vi "Path_Function_Deviation.vi"(10 "Function In":string, 11 "Path Points In":T1(array[cluster])) -> (3 "Path Points Out":T1(array[cluster]))   [LabVIEW 2019]
uses:
  <vilib>/gmath/NI_Gmath.lvlib
panel:
  out "X":dbl[][](graph)
  out "Y":dbl[][](graph)
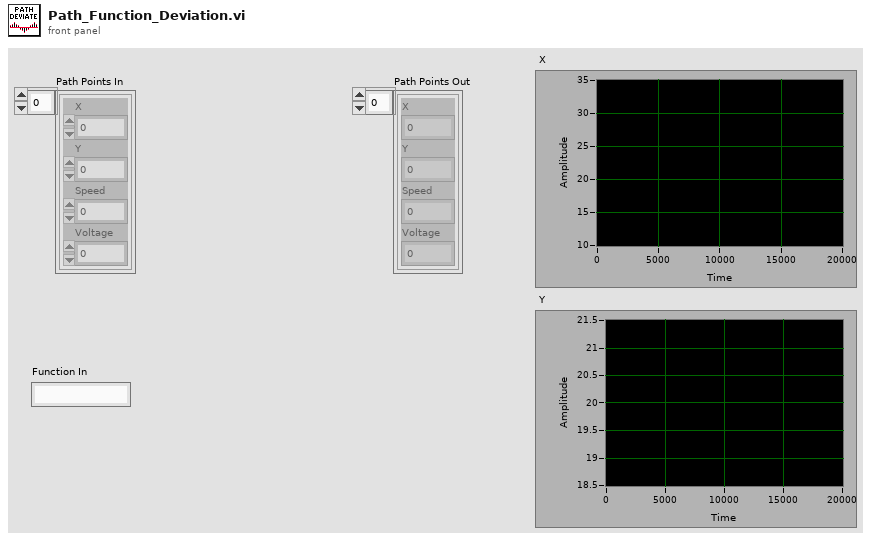
[diagram p1: front panel]
types:
  T1 = cluster{"X":dbl, "Y":dbl, "Speed":dbl, "Voltage":dbl}[]
  T2 = cluster{"X":dbl, "Y":dbl, "Speed":dbl, "Voltage":dbl}
  T3 = cluster{"X":bool, "Y":bool, "Speed":bool, "Voltage":bool}
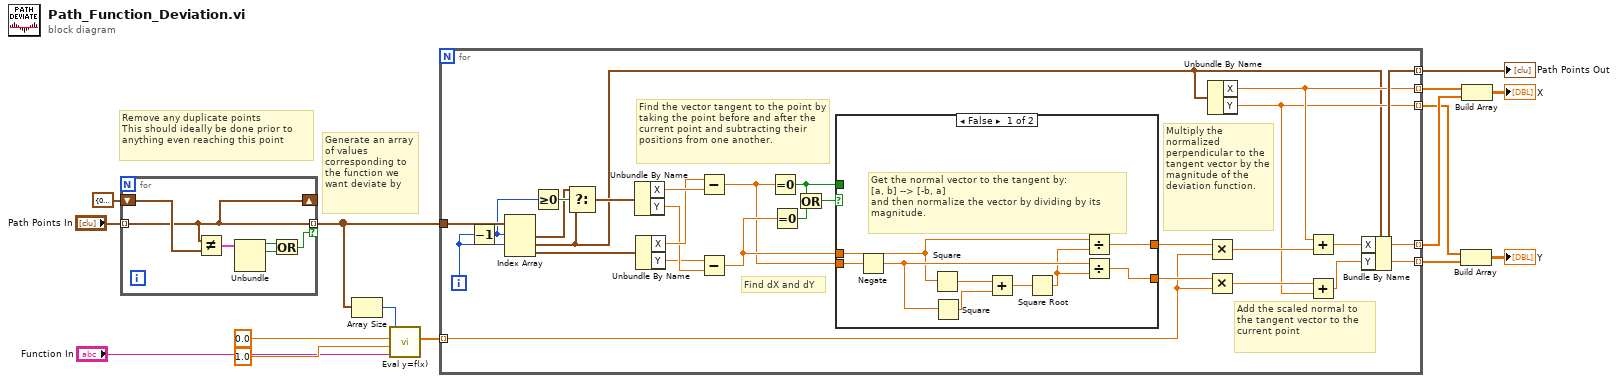
[diagram p0: block diagram]
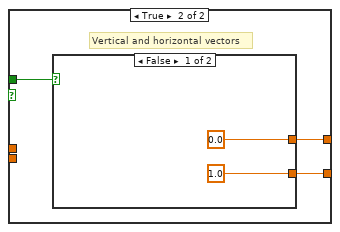
[diagram p2: hidden frame]
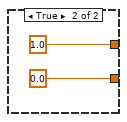
[diagram p3: hidden frame]
diagram:
  # "Generate an array of values corresponding to the function we want deviate by"
  # "Remove any duplicate points\nThis should ideally be done prior to anything even reaching this point"
  n1 = for {
    tunnel: "Path Points In" -> [w20] mode=indexing
    tunnel: [w20] -> w11 mode=indexing if=w16
    shift-right: [w20] -> _
    shift-left: T2 {"X"=0.0, "Y"=0.0, "Speed"=0.0, "Voltage"=0.0} ("Litho Point") -> [w21]
    n2 = Not Equal?(x=w20, y=w21) -> (x != y?=w19:T3)
    n3 = Unbundle(w19) -> ("X"=w18:bool, "Y"=w17:bool)  [unwired: 2 out]
    n4 = Or(x=w18, y=w17) -> (x .or. y?=w16:bool)
  }
  n5 = Array Size(array=w11) -> (size(s)=w14:i32)
  n6 = call <vilib>:"Eval y=f(x).vi"("formula"="Function In", "end"=1.0, "start"=0.0, "number of points"=w14) -> ("Y Values"=w12:dbl[])  [unwired: 3 out]
  n7 = for {
    tunnel: w11 -> [w48]
    tunnel: w12 -> [w32] mode=indexing
    tunnel: [w31] -> w7 mode=indexing
    tunnel: [w30] -> w4 mode=indexing
    tunnel: [w29] -> w2 mode=indexing
    tunnel: [w28] -> w3 mode=indexing
    tunnel: [w27] -> w1 mode=indexing
    i -> [w37]
    # "Add the scaled normal to the tangent vector to the current point"
    # "Multiply the normalized perpendicular to the tangent vector by the magnitude of the deviation function."
    # "Find the vector tangent to the point by taking the point before and after the current point and subtracting their positions from one another."
    # "Find dX and dY"
    n8 = Decrement(x=w37) -> (x-1=w26:i32)
    n9 = Index Array(array=w48, index #1=w26, index #2=w37) -> (element #1=w22:T2, element #2=w23:T2, element #3=w47:T2)  [unwired: 1 in]
    n10 = Greater Or Equal To 0?(x=w26) -> (x >= 0?=w25:bool)
    n11 = Select(t=w22, s=w25, f=w23) -> (s? t:f=w24:T2)
    n12 = Unbundle By Name(w24) -> ("X"=w46:dbl, "Y"=w44:dbl)
    n13 = Unbundle By Name(w47) -> ("X"=w45:dbl, "Y"=w43:dbl)
    n14 = Subtract(x=w45, y=w46) -> (x-y=w35:dbl)
    n15 = Subtract(x=w43, y=w44) -> (x-y=w36:dbl)
    n16 = Equal To 0?(x=w35) -> (x = 0?=w38:bool)
    n17 = Equal To 0?(x=w36) -> (x = 0?=w39:bool)
    n18 = Or(x=w38, y=w39) -> (x .or. y?=w40:bool)
    n19 = case shown="False" w40 {
      tunnel: [w50 w58] -> w33
      tunnel: [w56 w59] -> w34
      tunnel: w35 -> [w57 _]
      tunnel: w36 -> [w49 _]
      tunnel: w38 -> [_ w60]
      frame False {
        # "Get the normal vector to the tangent by:\n[a, b] --> [-b, a]\nand then normalize the vector by dividing by its magnitude."
        n20 = Negate(x=w57) -> (-x=w52:dbl)
        n21 = Square(x=w49) -> (x^2=w55:dbl)
        n22 = Square(x=w52) -> (x^2=w54:dbl)
        n23 = Add(x=w55, y=w54) -> (x+y=w53:dbl)
        n24 = Square Root(x=w53) -> (sqrt(x)=w51:dbl)
        n25 = Divide(x=w49, y=w51) -> (x/y=w56:dbl)
        n26 = Divide(x=w52, y=w51) -> (x/y=w50:dbl)
      }
      frame True {
        # "Vertical and horizontal vectors"
        n27 = case shown="False" w60 {
          tunnel: [0.0 1.0] -> w59
          tunnel: [1.0 0.0] -> w58
          frame False {
          }
          frame True {
          }
        }
      }
    }
    n28 = Multiply(x=w34, y=w32) -> (x*y=w41:dbl)
    n29 = Multiply(x=w33, y=w32) -> (x*y=w42:dbl)
    n30 = Unbundle By Name(w23) -> ("X"=w28:dbl, "Y"=w27:dbl)
    n31 = Add(x=w28, y=w41) -> (x+y=w29:dbl)
    n32 = Add(x=w42, y=w27) -> (x+y=w30:dbl)
    n33 = Bundle By Name(cluster=w23, "X"=w29, "Y"=w30) -> (w31:T2)
  }
  "Path Points Out" <- w7
  n34 = Build Array(w1, w4) -> (→"Y":dbl[][])
  n35 = Build Array(w3, w2) -> (→"X":dbl[][])
